vi "OAT Get DGT Window Boundaries.vi"(7 "offset":i32, 8 "dM":i32, 9 "actual window length":i32, 11 "# of Gabor windows":i32) -> (0 "start positions":i32[](array[numeric]), 1 "end positions":i32[](array[numeric]), 5 "next offset":i32)   [LabVIEW 2017, in "SoundVib_Gabor.lvlib"]
uses:
  <vilib>/addons/Sound and Vibration/Order Analysis/Gabor Order Tracking/SoundVib_Gabor.lvlib
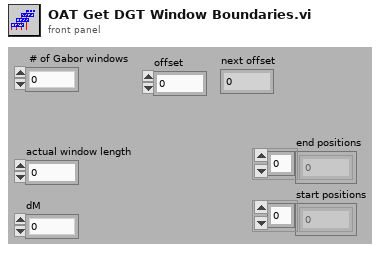
[diagram p1: front panel]
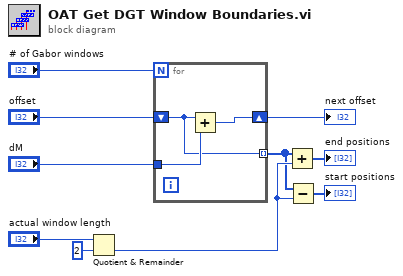
[diagram p0: block diagram]
diagram:
  n1 = Quotient & Remainder(x="actual window length", y=2) -> (floor(x/y)=w2:i32)  [unwired: 1 out]
  n2 = for {
    N: "# of Gabor windows" -> [_]
    shift-right: [w12] -> w8
    shift-left: "offset" -> [w11]
    tunnel: "dM" -> [w13]
    tunnel: [w11] -> w1 mode=indexing
    n3 = Add(x=w11, y=w13) -> (x+y=w12:i32)
  }
  "next offset" <- w8
  n4 = Add(x=w1, y=w2) -> (x+y=→"end positions":i32[])
  n5 = Subtract(x=w1, y=w2) -> (x-y=→"start positions":i32[])
